vi "test Execute Timeout.vi"(8 "error in (no error)":errorcluster, 11 "TestCase in":refnum<class "Single Consumer Test Case.lvclass">) -> (0 "error out":errorcluster, 3 "TestCase out":refnum<class "Single Consumer Test Case.lvclass">)   [LabVIEW 2017, in "Single Consumer Test Case.lvclass"]
uses:
  Single Consumer Test Case.lvclass
  Support/Messages/Test Message/Test Message.lvclass
  C:/github/niveristand-custom-device-message-library/Source/Message/Abstract Message/Abstract Message.lvclass
  Single Consumer Test Case.lvclass/Single Consumer Test Case.ctl
  Producer/Abstract Producer/Abstract Producer.lvclass
  <vilib>/addons/_JKI Toolkits/VI Tester/TestCase.llb/TestCase.lvclass
  Consumer/Abstract Consumer/Abstract Consumer.lvclass
  C:/Program Files (x86)/National Instruments/LabVIEW 2017/vi.lib/addons/_JKI Toolkits/VI Tester/TestCase.llb/TestCase.lvclass
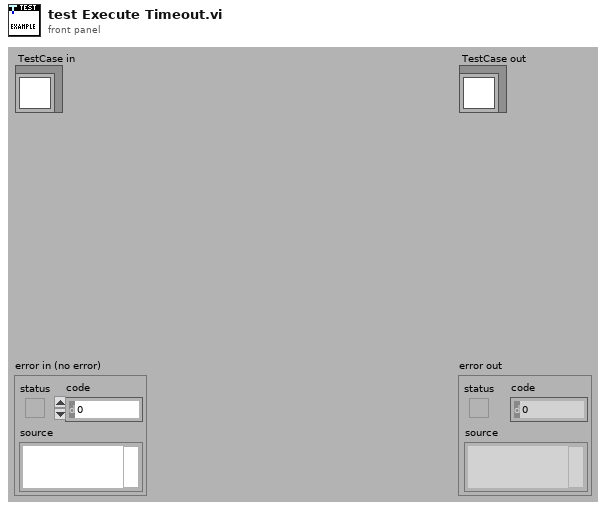
[diagram p1: front panel]
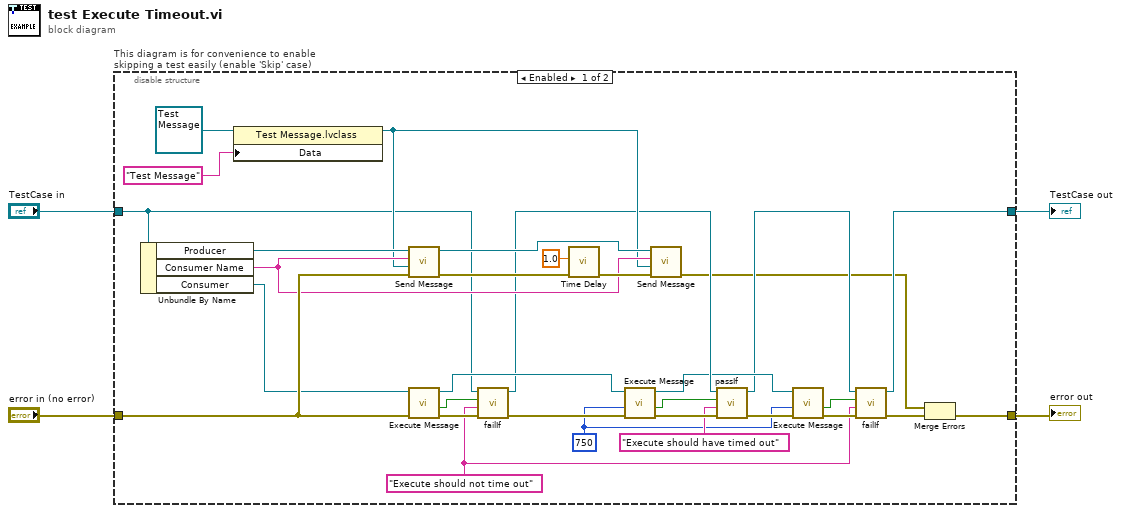
[diagram p0: block diagram]
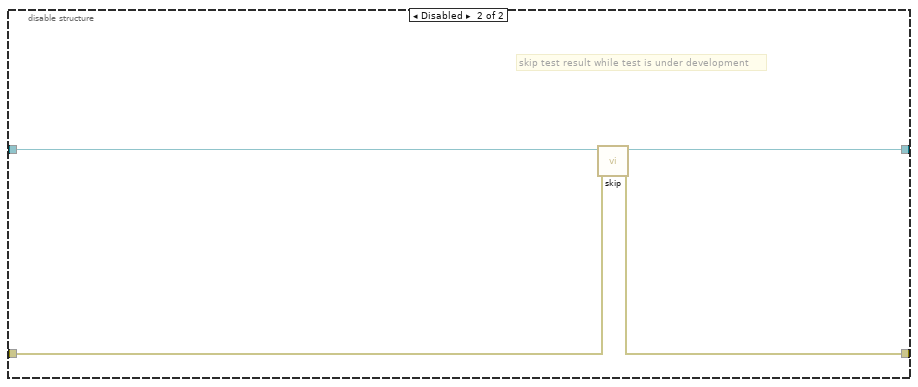
[diagram p2: hidden frame]
diagram:
  n1 = disable-structure "This diagram is for convenience to enable skipping a test easily (enable 'Skip' case)" shown="Enabled" {
    disable-tunnel: "TestCase in" -> [w22 w39]
    disable-tunnel: [w11 w37] -> w1
    disable-tunnel: [w5 w38] -> w3
    disable-tunnel: "error in (no error)" -> [w32 w36]
    frame Enabled {
      w8 = "Execute should not time out" ("message (\"\")")
      w13 = 750 ("timeout in ms (-1)")
      n2 = Unbundle By Name(w22) -> ("Producer"=w33:refnum<class "Abstract Producer.lvclass">, "Consumer Name"=w25:string, "Consumer"=w31:refnum<class "Abstract Consumer.lvclass">)
      n3 = property class="Test Message.lvclass"(reference=refnum<class "Test Message.lvclass"> refnum ("Test Message.lvclass"), "Data"="Test Message") -> (reference out=w24:refnum<class "Test Message.lvclass">)  [unwired: 1 in, 1 out]
      n4 = call-dynamic "Send Message.vi"("error in (no error)"=w32, "Message in"=w24, "Consumer in"=w25, "Abstract Producer in"=w33) -> ("error out"=w30:errorcluster, "Abstract Producer out"=w26:refnum<class "Abstract Producer.lvclass">)  [unwired: 4 in, 2 out]
      n5 = call "Execute Message.vi"("error in (no error)"=w32, "Abstract Consumer in"=w31) -> ("error out"=w21:errorcluster, "timed out?"=w23:bool, "Abstract Consumer out"=w29:refnum<class "Abstract Consumer.lvclass">)  [unwired: 6 in, 1 out]
      n6 = call-dynamic "failIf.vi"("error in (no error)"=w21, "message (\"\")"=w8, "fail"=w23, "TestCase in"=w22) -> ("error out"=w20:errorcluster, "TestCase out"=w18:refnum<class "Single Consumer Test Case.lvclass">)  [unwired: 6 in]
      n7 = call "Time Delay"("error in (no error)"=w30, "Delay Time (s)"=1.0) -> ("error out"=w27:errorcluster)  [unwired: 9 in]
      n8 = call "Execute Message.vi"("error in (no error)"=w20, "timeout in ms (-1)"=w13, "Abstract Consumer in"=w29) -> ("error out"=w19:errorcluster, "timed out?"=w17:bool, "Abstract Consumer out"=w15:refnum<class "Abstract Consumer.lvclass">)  [unwired: 5 in, 1 out]
      n9 = call-dynamic "Send Message.vi"("error in (no error)"=w27, "Message in"=w24, "Consumer in"=w25, "Abstract Producer in"=w26) -> ("error out"=w6:errorcluster)  [unwired: 4 in, 3 out]
      n10 = call-dynamic "passIf.vi"("error in (no error)"=w19, "message (\"\")"="Execute should have timed out" ("message (\"\")"), "pass"=w17, "TestCase in"=w18) -> ("error out"=w14:errorcluster, "TestCase out"=w12:refnum<class "Single Consumer Test Case.lvclass">)  [unwired: 6 in]
      n11 = call "Execute Message.vi"("error in (no error)"=w14, "timeout in ms (-1)"=w13, "Abstract Consumer in"=w15) -> ("error out"=w10:errorcluster, "timed out?"=w9:bool)  [unwired: 5 in, 2 out]
      n12 = call-dynamic "failIf.vi"("error in (no error)"=w10, "message (\"\")"=w8, "fail"=w9, "TestCase in"=w12) -> ("error out"=w7:errorcluster, "TestCase out"=w11:refnum<class "Single Consumer Test Case.lvclass">)  [unwired: 6 in]
      n13 = Merge Errors(w6, w7) -> (w5:errorcluster)
    }
    frame Disabled {
      # "skip test result while test is under development"
      n14 = call <vilib>:"skip.vi"("error in (no error)"=w36, "TestCase in"=w39) -> ("error out"=w38:errorcluster, "TestCase out"=w37:refnum<class "Single Consumer Test Case.lvclass">)  [unwired: 8 in]
    }
  }
  "error out" <- w3
  "TestCase out" <- w1
